vi "Read.vi"(8 "error in (no error)":errorcluster, 11 "U32 Array in":refnum<class "U32 Array.lvclass">) -> (0 "error out":errorcluster, 2 "U32 Array":u32[](array[numeric]), 3 "U32 Array out":refnum<class "U32 Array.lvclass">)   [LabVIEW 2020, in "Data.lvlib" / "U32 Array.lvclass"]
doc: "Read U32 Array."
uses:
  U32 Array.lvclass
  U32 Array.lvclass/U32 Array.ctl
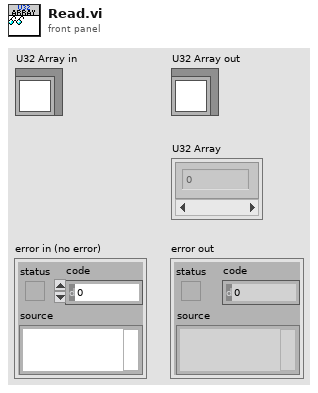
[diagram p1: front panel]
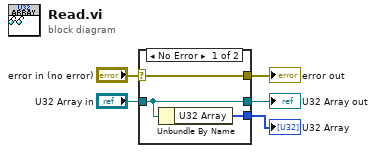
[diagram p0: block diagram]
diagram:
  n1 = case shown="No Error" "error in (no error)" {
    selector: "error in (no error)" -> [w8 w9]
    tunnel: [w8 w9] -> w4
    tunnel: [w7 w10] -> w2
    tunnel: "U32 Array in" -> [w7 w10]
    tunnel: [w6 _] -> w1
    frame No Error {
      n2 = Unbundle By Name(w7) -> ("U32 Array"=w6:u32[])
    }
    frame Error {
    }
  }
  "error out" <- w4
  "U32 Array out" <- w2
  "U32 Array" <- w1
